vi "Write Test Interval.vi"(8 "error in (no error)":errorcluster, 10 "Check Interval":u32, 11 "bt_Parallel_Threaded in":refnum<class "bt_Parallel_Threaded.lvclass">) -> (0 "error out":errorcluster, 3 "bt_Parallel_Threaded out":refnum<class "bt_Parallel_Threaded.lvclass">)   [LabVIEW 2021, in "BT.lvlib" / "bt_Parallel_Threaded.lvclass"]
uses:
  bt_Parallel_Threaded.lvclass
  bt_Parallel_Threaded.lvclass/bt_Parallel_Threaded.ctl
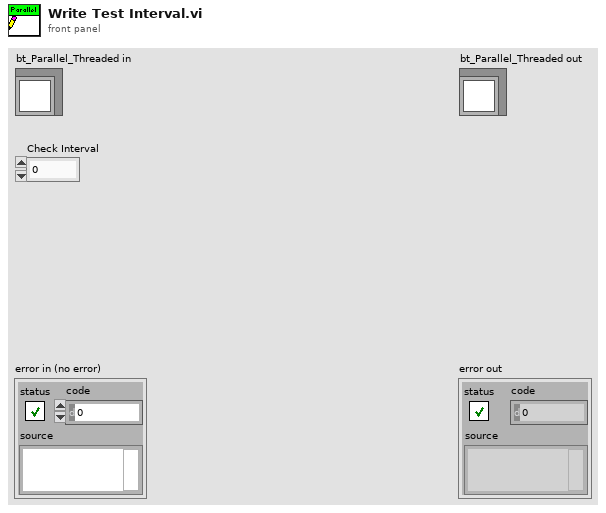
[diagram p1: front panel]
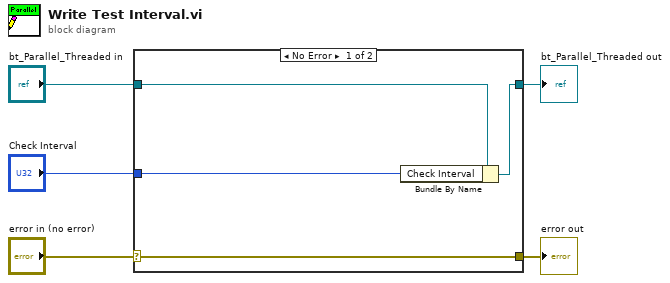
[diagram p0: block diagram]
diagram:
  n1 = case shown="No Error" "error in (no error)" {
    selector: "error in (no error)" -> [w9 w10]
    tunnel: [w9 w10] -> w4
    tunnel: [w7 w11] -> w2
    tunnel: "bt_Parallel_Threaded in" -> [w8 w11]
    tunnel: "Check Interval" -> [w6 _]
    frame No Error {
      n2 = Bundle By Name(cluster=w8, "Check Interval"=w6) -> (w7:refnum<class "bt_Parallel_Threaded.lvclass">)
    }
    frame Error {
    }
  }
  "error out" <- w4
  "bt_Parallel_Threaded out" <- w2
